vi "progra 4.vi"() -> ()   [LabVIEW 2011]
panel:
  out "?":bool
  out "80-120":bool
  out "1-80":bool
  out "Velocidad":dbl(knob) scale=0.0..180.0
  # "121-180"
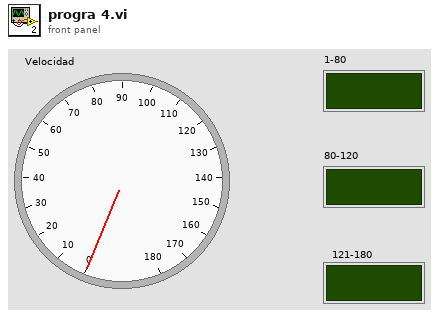
[diagram p1: front panel]
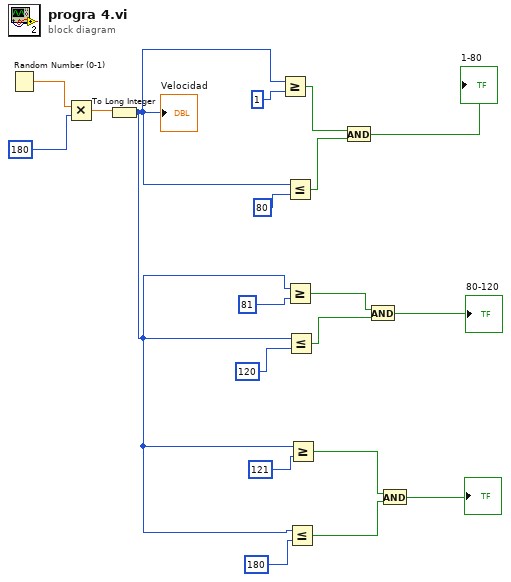
[diagram p0: block diagram]
diagram:
  n1 = Random Number (0-1)() -> (number: 0 to 1=w19:dbl)
  n2 = Multiply(x=w19, y=180) -> (x*y=w17:dbl)
  n3 = To Long Integer(number=w17) -> (32bit integer=w4:i32)
  "Velocidad" <- w4
  n4 = Greater Or Equal?(x=w4, y=1) -> (x >= y?=w13:bool)
  n5 = Less Or Equal?(x=w4, y=80) -> (x <= y?=w12:bool)
  n6 = Greater Or Equal?(x=w4, y=81) -> (x >= y?=w9:bool)
  n7 = Less Or Equal?(x=w4, y=120) -> (x <= y?=w8:bool)
  n8 = Less Or Equal?(x=w4, y=180) -> (x <= y?=w3:bool)
  n9 = Greater Or Equal?(x=w4, y=121) -> (x >= y?=w2:bool)
  n10 = And(x=w13, y=w12) -> (x .and. y?=→"1-80":bool)
  n11 = And(x=w9, y=w8) -> (x .and. y?=→"80-120":bool)
  n12 = And(x=w2, y=w3) -> (x .and. y?=→"?":bool)
